vi "ForceTimestamp.vi"(11 "In":waveform(dbl)[](array[waveform])) -> (3 "Out":waveform(dbl)[](array[waveform]))   [LabVIEW 2019]
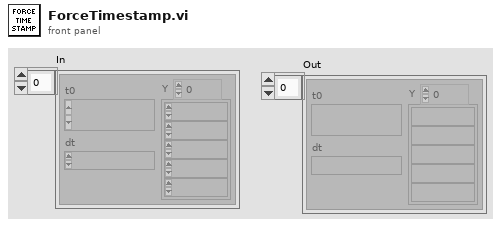
[diagram p1: front panel]
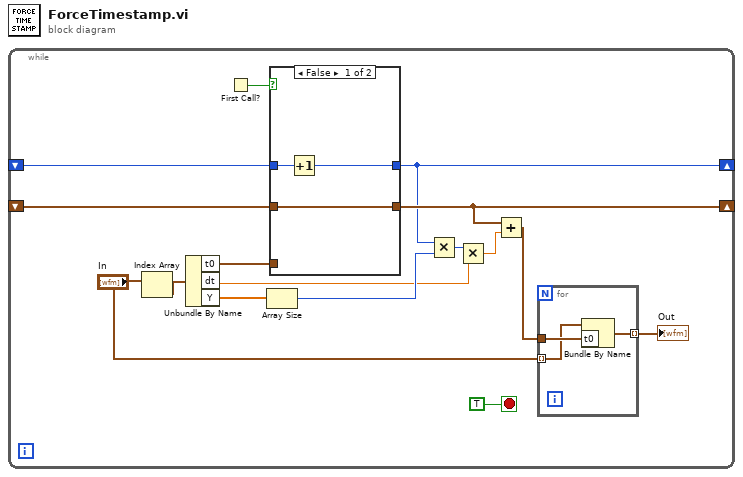
[diagram p0: block diagram]
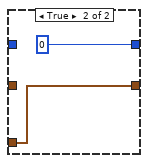
[diagram p2: hidden frame]
diagram:
  n1 = while {
    shift-right: [w11] -> _
    shift-left: _ -> [w13]
    shift-right: [w10] -> _
    shift-left: _ -> [w12]
    stop <- TRUE stop-if-true
    n2 = Index Array(array="In") -> (element=w3:waveform(dbl))  [unwired: 1 in]
    n3 = Unbundle By Name(w3) -> ("t0"=w15:timestamp, "dt"=w6:dbl, "Y"=w9:dbl[])
    n4 = First Call?() -> (First Call?: T/F=w14:bool)
    n5 = Array Size(array=w9) -> (size(s)=w8:i32)
    n6 = case shown="False" w14 {
      tunnel: w15 -> [_ w24]
      tunnel: w13 -> [w22 _]
      tunnel: [w22 w24] -> w11
      tunnel: [w21 0] -> w10
      tunnel: w12 -> [w20 _]
      frame False {
        n7 = Increment(x=w20) -> (x+1=w21:i32)
      }
      frame True {
      }
    }
    n8 = Multiply(x=w10, y=w8) -> (x*y=w7:i32)
    n9 = Multiply(x=w7, y=w6) -> (x*y=w5:dbl)
    n10 = Add(x=w11, y=w5) -> (x+y=w4:timestamp)
    n11 = for {
      tunnel: w4 -> [w19]
      tunnel: "In" -> [w18] mode=indexing
      tunnel: [w17] -> w1 mode=indexing
      n12 = Bundle By Name(cluster=w18, "t0"=w19) -> (w17:waveform(dbl))
    }
    "Out" <- w1
  }
